vi "Simple Proportional.vi"(1 "Proportionality Constant":dbl, 2 "Deadband":dbl, 3 "Current Value":dbl, 4 "Setpoint":dbl) -> (0 "Output":dbl)   [LabVIEW 2014]
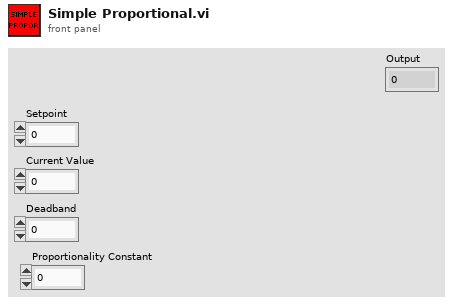
[diagram p1: front panel]
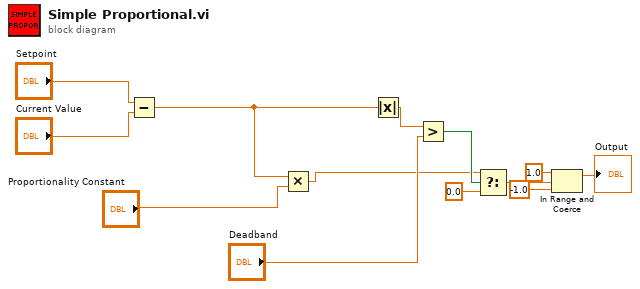
[diagram p0: block diagram]
diagram:
  n1 = Subtract(x="Setpoint", y="Current Value") -> (x-y=w10:dbl)
  n2 = Multiply(x=w10, y="Proportionality Constant") -> (x*y=w5:dbl)
  n3 = Absolute Value(x=w10) -> (abs(x)=w6:dbl)
  n4 = Greater?(x=w6, y="Deadband") -> (0:w8:bool)
  n5 = Select(t=w5, s=w8, f=0.0) -> (s? t:f=w3:dbl)
  n6 = In Range and Coerce(upper limit=1.0, x=w3, lower limit=-1.0) -> (coerced(x)=→"Output":dbl)  [unwired: 1 out]
